vi "isPlaying.vi"(8 "error in (no error)":errorcluster, 11 "Player in":refnum<class "Player.lvclass">) -> (0 "error out":errorcluster, 2 "playing":bool, 3 "Player out":refnum<class "Player.lvclass">)   [LabVIEW 2017, in "Player.lvclass"]
uses:
  Player.lvclass
  Player.lvclass/Player.ctl
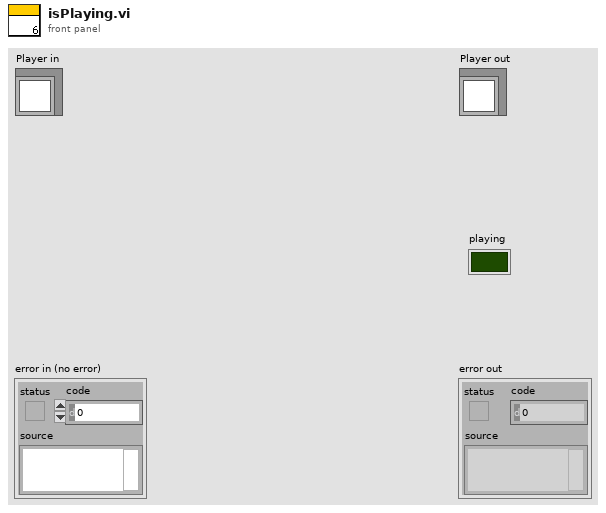
[diagram p1: front panel]
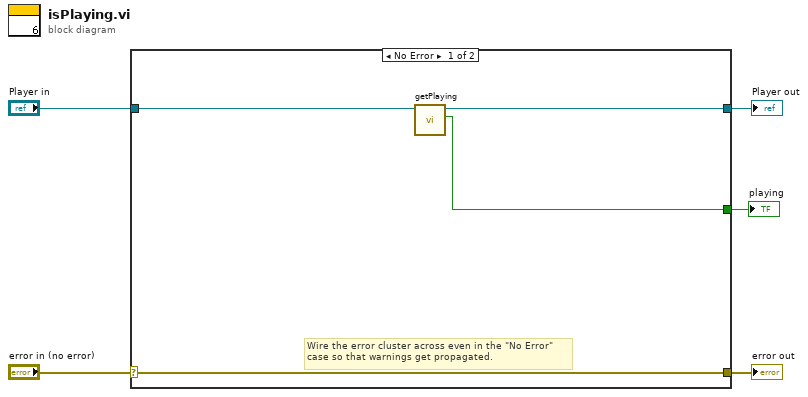
[diagram p0: block diagram]
diagram:
  n1 = case shown="No Error" "error in (no error)" {
    selector: "error in (no error)" -> [w8 w11]
    tunnel: [w8 w11] -> w4
    tunnel: [w7 w10] -> w2
    tunnel: "Player in" -> [w9 w10]
    tunnel: [w6 _] -> w1
    frame No Error {
      # "Wire the error cluster across even in the \"No Error\"\ncase so that warnings get propagated."
      n2 = call "getPlaying.vi"("Player in"=w9) -> ("playing"=w6:bool, "Player out"=w7:refnum<class "Player.lvclass">)  [unwired: 8 in, 1 out]
    }
    frame Error {
    }
  }
  "error out" <- w4
  "Player out" <- w2
  "playing" <- w1
